vi "MainV2.vi"() -> ()   [LabVIEW 2010]
uses:
  <vilib>/Instr/_visa.llb/VISA Set IO Buffer Mask.ctl
  <vilib>/Instr/_visa.llb/VISA Flush IO Buffer Mask.ctl
  GlobalVar.vi
  <vilib>/Instr/_visa.llb/VISA Configure Serial Port (Instr).vi
  <vilib>/Utility/file.llb/Write To Spreadsheet File (string).vi
panel:
  out "Index Tableau":i32
  out "sortie d'erreur 3":errorcluster caption="sortie d'erreur"
  out "sortie d'erreur 2":errorcluster caption="sortie d'erreur"
  out "sortie d'erreur":errorcluster
  in  "Send":bool
  in  "Data to send":sgl
  in  "Command type":u16(ring)=129 items=["COEF_COURANT_2_INF"=36, "COEF_COURANT_2_CON"=164, "COEF_COURANT_1_INF"=35, "COEF_COURANT_1_CON"=163, "COEF_HYSTERISIS_SECURITE_INF"=34, "POURCENT_SECURITE_MOTEUR_INF"=33, "VITESSE_TROTTOIR_MAX_INF"=32, "DEMARRAGE_DELAI_EQUILIBRE_INF"=31, "DEMARRAGE_TOL_GUIDON_INF"=30, "DEMARRAGE_TOL_ANGLE_INF"=29, "LIMITE_DISTANCE_UTILISATEUR_INF"=28, "GUIDONMAX_INF"=27, "ACCELERATION_COEF_FILTRE_INF"=26, "COEF_KALMAN_INF"=25, "PRINC_DIR_INF"=24, "PRINC_PID_D_INF"=23, "PRINC_PID_K_INF"=22, "COEF_HYSTERISIS_SECURITE_CON"=162, "POURCENT_SECURITE_MOTEUR_CON"=161, "VITESSE_TROTTOIR_MAX_CON"=160, "DEMARRAGE_DELAI_EQUILIBRE_CON"=159, "DEMARRAGE_TOL_GUIDON_CON"=158, "DEMARRAGE_TOL_ANGLE_CON"=157, "LIMITE_DISTANCE_UTILISATEUR_CON"=156, "GUIDONMAX_CON"=155, "ACCELERATION_COEF_FILTRE_CON"=154, "COEF_KALMAN_CON"=153, "PRINC_DIR_CON"=152, "PRINC_PID_D_CON"=151, "PRINC_PID_K_CON"=150, "ENREGISTER_DEMARRAGE"=149, "CHARGER_DEMARRAGE"=148, "ENREGISTRER_ASSERVISSEMENT"=147, "CHARGER_ASSERVISSEMENT"=146, "ENREGISTRER_VITESSE"=145, "CHARGER_VITESSE"=144, "DEMANDE_COEFFICIENTS"=137, "VERBOSE_INF"=8, "VERBOSE_CON"=136, "ETAT"=1, "STOP"=131, "DEPART"=130, "TEST_COM"=129]
  out "LongToSend":u8
  out "TypeToSend":u8
  out "DataToSend":u8[](array[numeric])
  out "Frequency":dbl
  out "Enum":T1(ring)
  out "error":errorcluster
  out "error Connexion":errorcluster
  out "Stop main loop":bool
  in  "stop":bool
  in  "Tab Control":T2(tab)
  out "Reception":string
  in  "Comm_BaudRate":u32=9600 caption="Baud rate"
  in  "Comm_PortComm":refnum<visa-resource-name>="COM33" caption="Communication Port"
  in  "timeout (10sec)":u32=10000
  in  "Con_RefreshIntensity":bool caption="Bouton OK 12"
  in  "Con_RefreshRightTorque":bool caption="Bouton OK 12"
  out "Con_XYIntensity":cluster{"Y":dbl[], "Y":dbl[]}[](graph) caption="Intensity"
  out "Con_XYRightTorque":cluster{"Y":dbl[], "Y":dbl[]}[](graph) caption="Motor right Torque"
  in  "Con_RefreshLeftTorque":bool caption="Bouton OK 12"
  out "Con_XYLeftTorque":cluster{"Y":dbl[], "Y":dbl[]}[](graph) caption="Motor left Torque"
  out "Con_IntensityMax":bool caption="Max Intensity"
  out "Con_Intensity":string[][](array[string]) caption="Intensity (A)"
  out "Con_MotorRightTorque":string[][](array[string]) caption="Motor right Torque (N.m)"
  out "Con_MotorLeftTorque":string[][](array[string]) caption="Motor left Torque (N.m)"
  in  "Ana_RefreshBattery":bool caption="Bouton OK 12"
  out "Ana_XYBattery":cluster{"Y":dbl[], "Y":dbl[]}[](graph) caption="Motor left Torque"
  in  "Ana_RefreshHandlebar":bool caption="Bouton OK 12"
  out "Ana_XYHandlebar":cluster{"Y":dbl[], "Y":dbl[]}[](graph) caption="Motor left Torque"
  out "Ana_Battery":string[][](array[string]) caption="Battery"
  out "Ana_Handlebar":string[][](array[string]) caption="Handlebar"
  in  "Inc_RefreshAcceleration":bool caption="Bouton OK 12"
  out "Inc_XYAcceleration":cluster{"Y":dbl[], "Y":dbl[]}[](graph) caption="Motor left Torque"
  in  "Inc_RefreshVelocityRightMotor":bool caption="Bouton OK 12"
  out "Inc_XYVelocityRightMotor":cluster{"Y":dbl[], "Y":dbl[]}[](graph) caption="Motor left Torque"
  in  "Inc_RefreshVelocityLeftMotor":bool caption="Bouton OK 12"
  out "Inc_XYVelocityLeftMotor":cluster{"Y":dbl[], "Y":dbl[]}[](graph) caption="Motor left Torque"
  out "Inc_Acceleration":string[][](array[string]) caption="Acceleration"
  out "Inc_VelocityRightMotor":string[][](array[string]) caption="Velocity Right motor"
  out "Inc_VelocityLeftMotor":string[][](array[string]) caption="Velocity left motor"
  out "Oth_XYAngularVelocity":cluster{"Y":dbl[], "Y":dbl[]}[](graph) caption="Motor left Torque"
  out "Oth_XYDistance":cluster{"Y":dbl[], "Y":dbl[]}[](graph) caption="Motor left Torque"
  out "Oth_XYAngle":cluster{"Y":dbl[], "Y":dbl[]}[](graph) caption="Motor left Torque"
  in  "Oth_RefreshAngularVelocity":bool caption="Bouton OK 12"
  in  "Oth_RefreshDistance":bool caption="Bouton OK 12"
  in  "Oth_RefreshAngle":bool caption="Bouton OK 12"
  out "Other_AngularVelocity":string[][](array[string]) caption="Angular velocity"
  out "Other_Distance":string[][](array[string]) caption="Distance"
  out "Other_Angle":string[][](array[string]) caption="Angle"
  in  "Analyse_Send":bool
  in  "Analyse_Time":dbl caption="Time"
  in  "Analyse_Step":dbl caption="Step"
  in  "Analyse_LeftOrRight":bool caption="Booléen"
  out "Analyse_XYTorque":cluster{"Y":dbl[], "Y":dbl[]}[](graph) caption="Motor Torque command"
  out "Analyse_MotorTorque":string[][](array[string]) caption="Motor  Torque (N.m)"
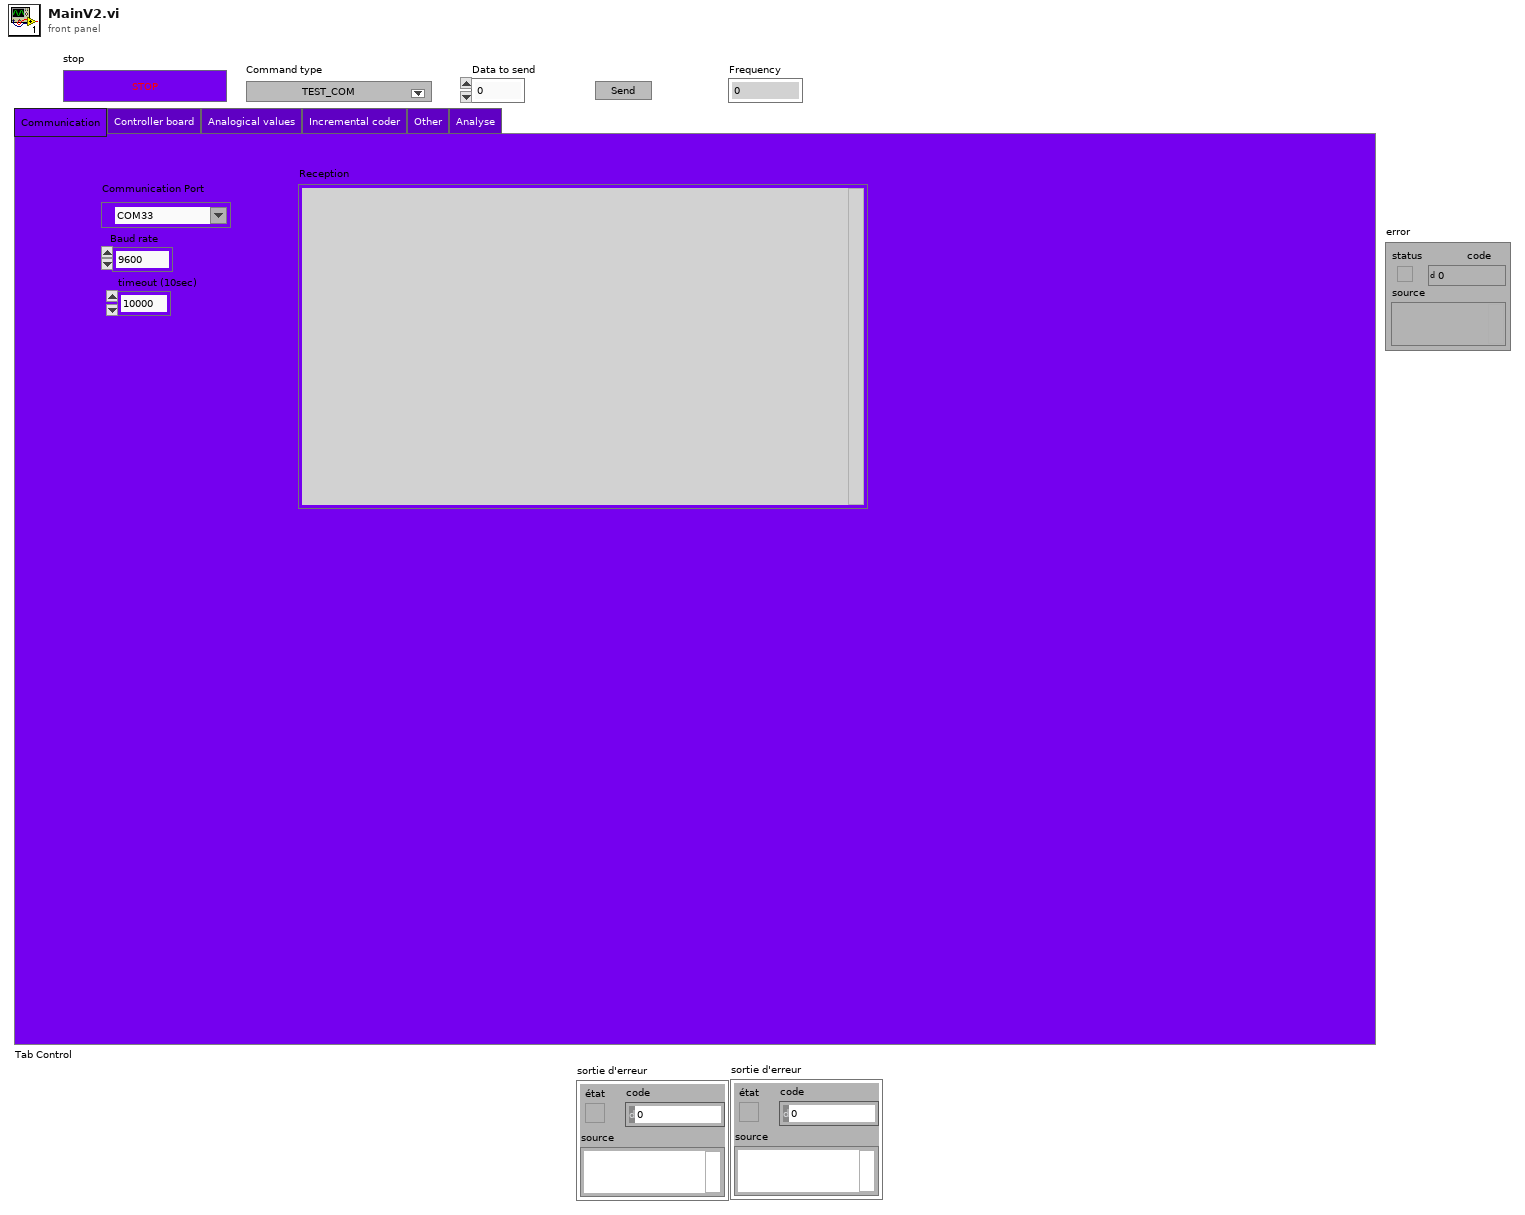
[diagram p1: front panel]
types:
  T1 = enum16{"Send_Instruction", "Con_RefreshLeftTorque", "Con_RefreshRightTorque", "Con_RefreshIntensity", "Ana_RefreshBattery", "Ana_RefreshHandlebar", "Inc_RefreshVelocityLeftMotor", "Inc_RefreshVelocityRightMotor", "Inc_RefreshAcceleration", "SendAnalysis", "Oth_RefreshAngle", "Oth_RefreshDistance", "Oth_RefreshAngularVelocity", "Waiting"}
  T2 = enum32{"Communication", "Controller board", "Analogical values", "Incremental coder", "Other", "Analyse"}
  T3 = typedef "VISA Set IO Buffer Mask.ctl" = u16
  T4 = typedef "VISA Flush IO Buffer Mask.ctl" = u16
  T5 = enum16{"Send_Instruction", "Con_RefreshLeftTorque", "Con_RefreshRightTorque", "Con_RefreshIntensity", "Ana_RefreshBattery", "Ana_RefreshHandlebar", "Inc_RefreshVelocityLeftMotor", "Inc_RefreshVelocityRightMotor", "Inc_RefreshAcceleration", "SendAnalysis", "Oth_RefreshAngle", "Oth_RefreshDistance", "Oth_RefreshAgularVelocity", "Waiting"}
  T6 = enum16{"Send_Instruction", "Con_RefreshLeftTorque", "Con_RefreshRightTorque", "Con_RefreshIntensity", "Ana_RefreshBattery", "Ana_RefreshHandlebar", "Inc_RefreshVelocityLeftMotor", "Inc_RefreshVelocityRightMotor", "Inc_RefreshAcceleration", "SendAnalysis", "Waiting"}
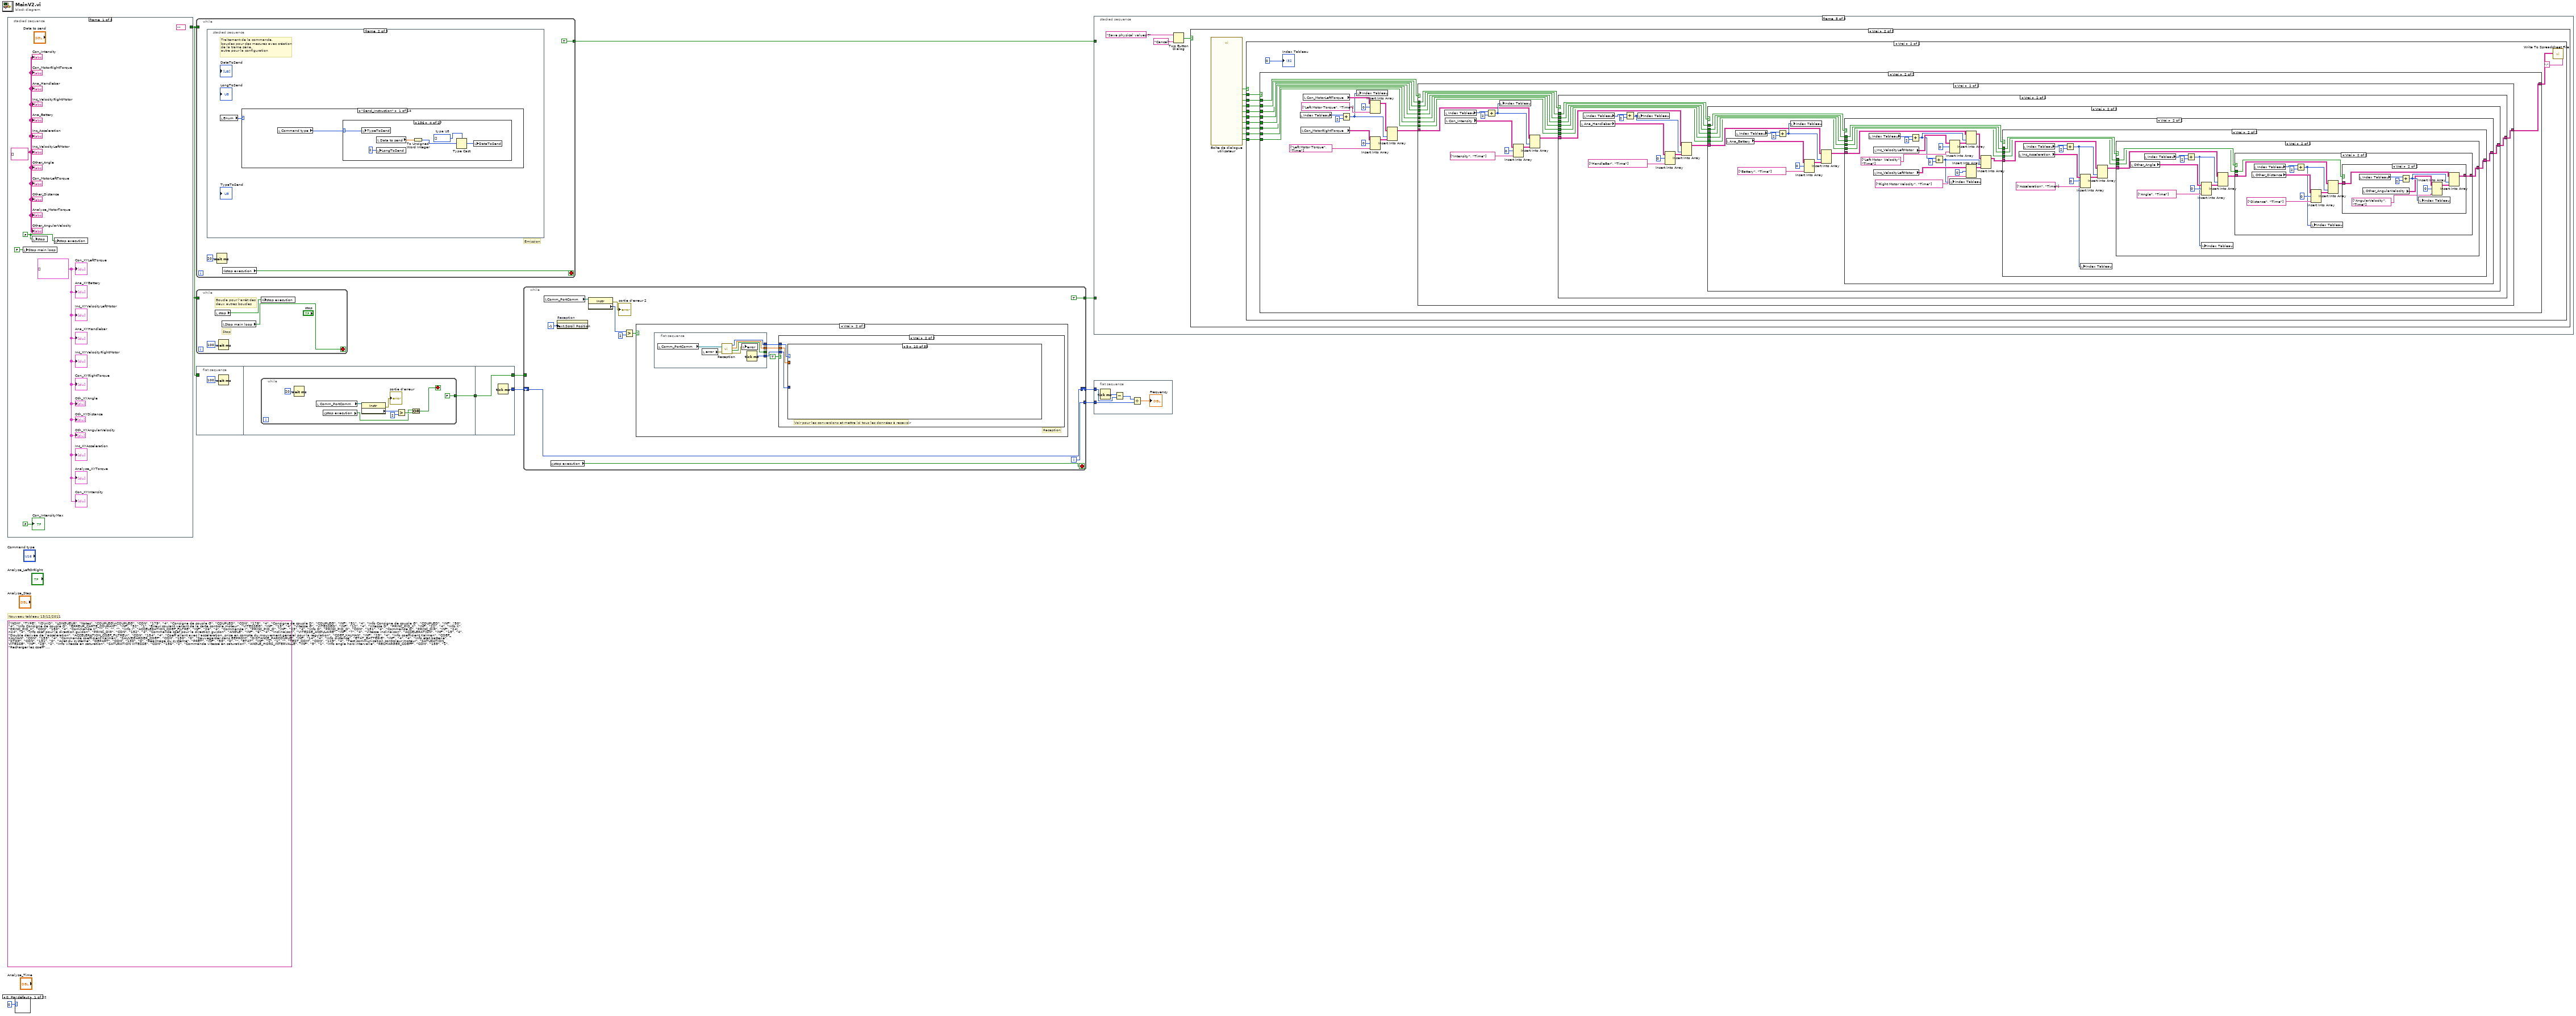
[diagram p0: block diagram]
diagram:
  (unwired) string[][] [["NOM", "TYPE", "ID\nID", "LONGUEUR", "Notes"], ["COUPLEG\nCOUPLEG", "CON", "179", "4", "Consigne de couple G"], ["COUPLED", "CON", "178", "4", "Consigne de couple D"], ["COUPLEG", "INF", "51", "4", "Info Consigne de couple G"], ["COUPLED", "INF", "50", "4", "Info Consigne de couple D"], ["ERREUR_CARTE_COURANT", "INF", "52", "1", "Erreur courant venant de la carte contrôle moteur"], ["VITESSEG", "INF", "13", "4", "Vitesse G"], ["VITESSED", "INF", "12", "4", "Vitesse D"], ["PRINC_PID_K", "INF", "22", "4", "Info K"], ["PRINC_PID_K", "CON", "150", "4", "Commande K"], ["", "", "", "", "Info I"], ["ACCELERATION_COEF_FILTRE", "INF", "26", "4", "Commande I"], ["PRINC_PID_D", "INF", "23", "4", "Info D"], ["PRINC_PID_D", "CON", "151", "4", "Commande D"], ["PRINC_DIR", "INF", "24\n24", "4", "Info coef pour la direction guidon"], ["PRINC_DIR", "CON", "152", "4", "Commande coef pour la direction guidon"], ["ANGLE", "INF", "6", "4", "Inclinaison"], ["VITESSE_ANGULAIRE", "INF", "7", "4", "Vitesse inclinaison"], ["ACCELERATION", "INF", "15", "4", "Double dérivée de l'accélération"], ["ACCELERATION_COEF_FILTRE\n", "CON", "154", "4", "Coeff allant avec l'accélération, prise en compte du mouvement général pour la régulation"], ["COEF_KALMAN", "INF", "25", "4", "Info coefficient Kalman"], ["COEF_KALMAN", "CON", "153", "4", "Commande coefficient Kalman"], ["SAUVEGARDER_COEF", "CON", "150", "0", "Sauvegarder dans EEPROM"], ["DISTANCE_PARCOURUE", "INF", "14", "4", "Info distance"], ["ETAT_BATTERIE", "INF", "4", "4", "Info etat batterie"], ["STOP", "CON", "131", "0", "Arret du système"], ["DEPART", "CON", "130", "0", "Réarmage du système"], ["PRET", "INF", "53", "0", ""], ["ETAT", "INF", "1", "1", ""], ["TEST_COM", "CON", "129", "4", "Test communication controleur moteur"], ["SATURATION_VITESSE", "INF", "28", "2", "Info vitesse en saturation"], ["SATURATION VITESSE", "CON", "156", "2", "Commande vitesse en saturation"], ["ANGLE_HORS_INTERVALLE", "INF", "5", "1", "Info angle hors intervalle"], ["RECHARGER_COEFF", "CON", "159", "1", "Recharger les coeff"], ["VERBOSE", "INF", "8", "2", ""], ["VERBOSE", "CON", "136", "2", ""], ["DEMANDE_COEFFICIENTS", "CON", "137", "1", ""], ["CHARGER_VITESSE", "CON", "144", "0", ""], ["ENREGISTRER_VITESSE", "CON", "145", "0", ""], ["CHARGER_ASSERVISSEMENT", "CON", "146", "0", ""], ["ENREGISTRER_ASSERVISSEMENT", "CON", "147", "0", ""], ["CHARGER_DEMARRAGE", "CON", "148", "0", ""], ["ENREGISTRER_DEMARRAGE", "CON", "149", "0", ""], ["GUIDONMAX", "INF", "27", "4", ""], ["LIMITE_DISTANCE_UTILISATEUR", "INF", "28", "4", ""], ["DEMARRAGE_TOL_ANGLE", "INF", "29", "4", ""], ["DEMARRAGE_TOL_GUIDON", "INF", "30", "4", ""], ["DEMARRAGE_DELAI_EQUILIBRE", "INF", "31", "4", ""], ["VITESSE_TROTTOIR_MAX", "INF", "32", "4", ""], ["POURCENT_SECURITE_MOTEUR", "INF", "33", "4", ""], ["COEF_HYSTERESIS_SECURITE", "INF", "34", "4", ""], ["COEF_COURANT_1", "CON", "163", "4", ""], ["COEF_COURANT_1", "INF", "35", "4", ""], ["COEF_COURANT_2", "CON", "164", "4", ""], ["COEF_COURANT_2", "INF", "36", "4", ""]]
  # "Nouveau tableau 13/12/2011"
  n1 = stacked-sequence {
    tunnel: [_ _ TRUE] -> w4
    frame #0 {
      (unwired) "" ("Spe_Liste")
      w11 = cluster{"Y":dbl[], "Y":dbl[]}[] [] ("Ana_XYHandlebar 3")
      w10 = string[][] [] ("Velocity motor left")
      w13 = FALSE ("Comm_LEDTest")
      n2 = local write "Stop main loop"(FALSE ("Stop main loop")) -> ()
      n3 = local write "stop"(w13) -> ()
      n4 = global write "GlobalVar.vi" "stop execution"(w13) -> ()
      "Con_IntensityMax" <- FALSE ("Con_IntensityMax")
      "Inc_Acceleration" <- w10
      "Other_Angle" <- w10
      "Other_Distance" <- w10
      "Ana_XYHandlebar" <- w11
      "Ana_XYBattery" <- w11
      "Inc_XYVelocityLeftMotor" <- w11
      "Inc_XYVelocityRightMotor" <- w11
      "Inc_XYAcceleration" <- w11
      "Con_MotorLeftTorque" <- w10
      "Con_MotorRightTorque" <- w10
      "Con_Intensity" <- w10
      "Inc_VelocityLeftMotor" <- w10
      "Inc_VelocityRightMotor" <- w10
      "Ana_Handlebar" <- w10
      "Ana_Battery" <- w10
      "Con_XYRightTorque" <- w11
      "Con_XYIntensity" <- w11
      "Con_XYLeftTorque" <- w11
      "Other_AngularVelocity" <- w10
      "Oth_XYAngle" <- w11
      "Oth_XYDistance" <- w11
      "Oth_XYAngularVelocity" <- w11
      "Analyse_XYTorque" <- w11
      "Analyse_MotorTorque" <- w10
    }
    frame #1 {
      w18 = T3 48 items=["Buffer d'entrées (E/S)"=16, "Buffer de sorties (E/S)"=32, "Buffer d'entrées et de sorties (E/S)"=48] ("Mask")
      w22 = T4 16 items=["Vider le buffer d'entrées"=16, "Écrire le buffer de sorties sur le périphérique"=32, "Vider le buffer d'entrées (Pas d'E/S)"=64, "Vider le buffer de sorties"=128] ("Mask")
      w25 = u16 0 items=["None"=0, "XON/XOFF"=1, "RTS/CTS"=2, "DTR/DSR"=4] ("flow control")
      w26 = u16 10 items=["1.0"=10, "1.5"=15, "2.0"=20] ("stop bits")
      w28 = u16 0 items=["None", "Odd", "Even", "Mark", "Space"] ("parity")
      # "Initial"
      n5 = local write "Tab Control"(T2."Communication" ("Tab Control")) -> ()
      n6 = call-poly "VISA Configure Serial Port"("VISA resource name"="Comm_PortComm", "timeout (10sec)"="timeout (10sec)", "baud rate (9600)"="Comm_BaudRate", "data bits (8)"=u16 8 ("data bits"), "parity (0:none)"=w28, "stop bits (10: 1 bit)"=w26, "flow control (0:none)"=w25) -> ("VISA resource name out"=w23:refnum<visa-resource-name>, "error out"=w20:errorcluster)  [unwired: 2 in, 5 out]
      "error Connexion" <- w20
      "error" <- w20
      n7 = VISA Set I/O Buffer Size(VISA resource name=w23, mask (16)=w18, size (4096)=u32 524288 ("taille (4096)"), error in (no error)=w20) -> (VISA resource name out=w21:refnum<visa-resource-name>, error out=w19:errorcluster)
      n8 = VISA Flush I/O Buffer(VISA resource name=w21, mask (16)=w22, error in (no error)=w19) -> ()  [unwired: 2 out]
      "Reception" <- "" ("Reception")
    }
    frame #2 {
      # "OK Initialisation"
    }
  }
  n9 = case shown="0, Par défaut" 0 {
    frame 0, Default {
    }
    frame 10 {
    }
    frame 11 {
    }
    frame 12 {
    }
    frame 13 {
    }
    frame 14 {
    }
    frame 15 {
    }
    frame 16 {
    }
    frame 17 {
    }
    frame 18 {
    }
    frame 19 {
    }
    frame 20 {
    }
    frame 21 {
    }
    frame 22 {
    }
    frame 23 {
    }
    frame 24 {
    }
    frame 25 {
    }
    frame 26 {
    }
    frame 27 {
    }
    frame 28 {
    }
    frame 29 {
    }
    frame 30 {
    }
  }
  n10 = while {
    tunnel: w4 -> [_]
    tunnel: [TRUE] -> w8
    stop <- w33 stop-if-true
    # "Emission"
    n11 = stacked-sequence {
      frame #0 {
        # "Detection de la commande\ndemandée"
        n12 = Build Array("Send", "Con_RefreshLeftTorque", "Con_RefreshRightTorque", "Con_RefreshIntensity", "Ana_RefreshBattery", "Ana_RefreshHandlebar", "Inc_RefreshVelocityLeftMotor", "Inc_RefreshVelocityRightMotor", "Inc_RefreshAcceleration", "Analyse_Send", "Oth_RefreshAngle", "Oth_RefreshDistance", "Oth_RefreshAngularVelocity") -> (w53:bool[])
        n13 = Search 1D Array(1D array=w53, element=TRUE) -> (index of element=w49:i32)  [unwired: 1 in]
        n14 = Equal?(x=w49, y=-1) -> (x = y?=w51:bool)
        n15 = case shown="Vrai" w51 {
          tunnel: [w54 T5."Waiting" ("Enum 2")] -> w50
          tunnel: w49 -> [w54 _]
          frame False {
          }
          frame True {
          }
        }
        "Enum" <- w50
      }
      frame #1 {
        # "Traitement de la commande,\nboucles pour des mesures avec création \nde la trame série,\nautre pour la configuration"
        n16 = local read "Enum"() -> (w56:T1)
        n17 = case shown="\"Send_Instruction\"" w56 {
          frame "Send_Instruction" {
            n18 = local read "Command type"() -> (w57:u16)
            n19 = case shown="136" w57 {
              selector: w57 -> [w62 w64 w69 w75 w79 w84 w89 w94 w99 w104 w109 w114 w119 w124 w129 w134 w139 w144 w149 w154 w159 w164 w169 w174 w179 w184 _]
              frame 129 {
                w60 = u8[] []  # type U8
                n20 = local write "TypeToSend"(w62) -> ()
                n21 = local write "LongToSend"(u8 4 ("LongToSend")) -> ()
                n22 = local read "Data to send"() -> (w58:sgl)
                n23 = Type Cast(type=w60, x=w58) -> (*(type *) &x=w59:u8[])
                n24 = local write "DataToSend"(w59) -> ()
              }
              frame 130 {
                w66 = u8[] []  # type U8
                n25 = local write "TypeToSend"(w64) -> ()
                n26 = local write "LongToSend"(u8 0 ("LongToSend")) -> ()
                n27 = local read "Data to send"() -> (w63:sgl)
                n28 = Type Cast(type=w66, x=w63) -> (*(type *) &x=w65:u8[])
                n29 = local write "DataToSend"(w65) -> ()
              }
              frame 131 {
                w71 = u8[] []  # type U8
                n30 = local write "TypeToSend"(w69) -> ()
                n31 = local write "LongToSend"(u8 0 ("LongToSend")) -> ()
                n32 = local read "Data to send"() -> (w68:sgl)
                n33 = Type Cast(type=w71, x=w68) -> (*(type *) &x=w70:u8[])
                n34 = local write "DataToSend"(w70) -> ()
              }
              frame 136 {
                w77 = u8[] []  # type U8
                n35 = local write "TypeToSend"(w75) -> ()
                n36 = local write "LongToSend"(u8 2 ("LongToSend")) -> ()
                n37 = local read "Data to send"() -> (w74:sgl)
                n38 = To Unsigned Word Integer(number=w74) -> (unsigned 16bit integer=w73:u16)
                n39 = Type Cast(type=w77, x=w73) -> (*(type *) &x=w76:u8[])
                n40 = local write "DataToSend"(w76) -> ()
              }
              frame 137 {
                w81 = u8[] []  # type U8
                n41 = local write "TypeToSend"(w79) -> ()
                n42 = local write "LongToSend"(u8 0 ("LongToSend")) -> ()
                n43 = local read "Data to send"() -> (w83:sgl)
                n44 = Type Cast(type=w81, x=w83) -> (*(type *) &x=w80:u8[])
                n45 = local write "DataToSend"(w80) -> ()
              }
              frame 144 {
                w86 = u8[] []  # type U8
                n46 = local write "TypeToSend"(w84) -> ()
                n47 = local write "LongToSend"(u8 0 ("LongToSend")) -> ()
                n48 = local read "Data to send"() -> (w88:sgl)
                n49 = Type Cast(type=w86, x=w88) -> (*(type *) &x=w85:u8[])
                n50 = local write "DataToSend"(w85) -> ()
              }
              frame 145 {
                w91 = u8[] []  # type U8
                n51 = local write "TypeToSend"(w89) -> ()
                n52 = local write "LongToSend"(u8 0 ("LongToSend")) -> ()
                n53 = local read "Data to send"() -> (w93:sgl)
                n54 = Type Cast(type=w91, x=w93) -> (*(type *) &x=w90:u8[])
                n55 = local write "DataToSend"(w90) -> ()
              }
              frame 146 {
                w96 = u8[] []  # type U8
                n56 = local write "TypeToSend"(w94) -> ()
                n57 = local write "LongToSend"(u8 0 ("LongToSend")) -> ()
                n58 = local read "Data to send"() -> (w98:sgl)
                n59 = Type Cast(type=w96, x=w98) -> (*(type *) &x=w95:u8[])
                n60 = local write "DataToSend"(w95) -> ()
              }
              frame 147 {
                w101 = u8[] []  # type U8
                n61 = local write "TypeToSend"(w99) -> ()
                n62 = local write "LongToSend"(u8 0 ("LongToSend")) -> ()
                n63 = local read "Data to send"() -> (w103:sgl)
                n64 = Type Cast(type=w101, x=w103) -> (*(type *) &x=w100:u8[])
                n65 = local write "DataToSend"(w100) -> ()
              }
              frame 148 {
                w106 = u8[] []  # type U8
                n66 = local write "TypeToSend"(w104) -> ()
                n67 = local write "LongToSend"(u8 0 ("LongToSend")) -> ()
                n68 = local read "Data to send"() -> (w108:sgl)
                n69 = Type Cast(type=w106, x=w108) -> (*(type *) &x=w105:u8[])
                n70 = local write "DataToSend"(w105) -> ()
              }
              frame 149 {
                w111 = u8[] []  # type U8
                n71 = local write "TypeToSend"(w109) -> ()
                n72 = local write "LongToSend"(u8 0 ("LongToSend")) -> ()
                n73 = local read "Data to send"() -> (w113:sgl)
                n74 = Type Cast(type=w111, x=w113) -> (*(type *) &x=w110:u8[])
                n75 = local write "DataToSend"(w110) -> ()
              }
              frame 150 {
                w116 = u8[] []  # type U8
                n76 = local write "TypeToSend"(w114) -> ()
                n77 = local write "LongToSend"(u8 4 ("LongToSend")) -> ()
                n78 = local read "Data to send"() -> (w118:sgl)
                n79 = Type Cast(type=w116, x=w118) -> (*(type *) &x=w115:u8[])
                n80 = local write "DataToSend"(w115) -> ()
              }
              frame 151 {
                w121 = u8[] []  # type U8
                n81 = local write "TypeToSend"(w119) -> ()
                n82 = local write "LongToSend"(u8 4 ("LongToSend")) -> ()
                n83 = local read "Data to send"() -> (w123:sgl)
                n84 = Type Cast(type=w121, x=w123) -> (*(type *) &x=w120:u8[])
                n85 = local write "DataToSend"(w120) -> ()
              }
              frame 152 {
                w126 = u8[] []  # type U8
                n86 = local write "TypeToSend"(w124) -> ()
                n87 = local write "LongToSend"(u8 4 ("LongToSend")) -> ()
                n88 = local read "Data to send"() -> (w128:sgl)
                n89 = Type Cast(type=w126, x=w128) -> (*(type *) &x=w125:u8[])
                n90 = local write "DataToSend"(w125) -> ()
              }
              frame 153 {
                w131 = u8[] []  # type U8
                n91 = local write "TypeToSend"(w129) -> ()
                n92 = local write "LongToSend"(u8 4 ("LongToSend")) -> ()
                n93 = local read "Data to send"() -> (w133:sgl)
                n94 = Type Cast(type=w131, x=w133) -> (*(type *) &x=w130:u8[])
                n95 = local write "DataToSend"(w130) -> ()
              }
              frame 154 {
                w136 = u8[] []  # type U8
                n96 = local write "TypeToSend"(w134) -> ()
                n97 = local write "LongToSend"(u8 4 ("LongToSend")) -> ()
                n98 = local read "Data to send"() -> (w138:sgl)
                n99 = Type Cast(type=w136, x=w138) -> (*(type *) &x=w135:u8[])
                n100 = local write "DataToSend"(w135) -> ()
              }
              frame 155 {
                w141 = u8[] []  # type U8
                n101 = local write "TypeToSend"(w139) -> ()
                n102 = local write "LongToSend"(u8 4 ("LongToSend")) -> ()
                n103 = local read "Data to send"() -> (w143:sgl)
                n104 = Type Cast(type=w141, x=w143) -> (*(type *) &x=w140:u8[])
                n105 = local write "DataToSend"(w140) -> ()
              }
              frame 156 {
                w146 = u8[] []  # type U8
                n106 = local write "TypeToSend"(w144) -> ()
                n107 = local write "LongToSend"(u8 4 ("LongToSend")) -> ()
                n108 = local read "Data to send"() -> (w148:sgl)
                n109 = Type Cast(type=w146, x=w148) -> (*(type *) &x=w145:u8[])
                n110 = local write "DataToSend"(w145) -> ()
              }
              frame 157 {
                w151 = u8[] []  # type U8
                n111 = local write "TypeToSend"(w149) -> ()
                n112 = local write "LongToSend"(u8 4 ("LongToSend")) -> ()
                n113 = local read "Data to send"() -> (w153:sgl)
                n114 = Type Cast(type=w151, x=w153) -> (*(type *) &x=w150:u8[])
                n115 = local write "DataToSend"(w150) -> ()
              }
              frame 158 {
                w156 = u8[] []  # type U8
                n116 = local write "TypeToSend"(w154) -> ()
                n117 = local write "LongToSend"(u8 4 ("LongToSend")) -> ()
                n118 = local read "Data to send"() -> (w158:sgl)
                n119 = Type Cast(type=w156, x=w158) -> (*(type *) &x=w155:u8[])
                n120 = local write "DataToSend"(w155) -> ()
              }
              frame 159 {
                w161 = u8[] []  # type U8
                n121 = local write "TypeToSend"(w159) -> ()
                n122 = local write "LongToSend"(u8 4 ("LongToSend")) -> ()
                n123 = local read "Data to send"() -> (w163:sgl)
                n124 = Type Cast(type=w161, x=w163) -> (*(type *) &x=w160:u8[])
                n125 = local write "DataToSend"(w160) -> ()
              }
              frame 160 {
                w166 = u8[] []  # type U8
                n126 = local write "TypeToSend"(w164) -> ()
                n127 = local write "LongToSend"(u8 4 ("LongToSend")) -> ()
                n128 = local read "Data to send"() -> (w168:sgl)
                n129 = Type Cast(type=w166, x=w168) -> (*(type *) &x=w165:u8[])
                n130 = local write "DataToSend"(w165) -> ()
              }
              frame 161 {
                w171 = u8[] []  # type U8
                n131 = local write "TypeToSend"(w169) -> ()
                n132 = local write "LongToSend"(u8 4 ("LongToSend")) -> ()
                n133 = local read "Data to send"() -> (w173:sgl)
                n134 = Type Cast(type=w171, x=w173) -> (*(type *) &x=w170:u8[])
                n135 = local write "DataToSend"(w170) -> ()
              }
              frame 162 {
                w176 = u8[] []  # type U8
                n136 = local write "TypeToSend"(w174) -> ()
                n137 = local write "LongToSend"(u8 4 ("LongToSend")) -> ()
                n138 = local read "Data to send"() -> (w178:sgl)
                n139 = Type Cast(type=w176, x=w178) -> (*(type *) &x=w175:u8[])
                n140 = local write "DataToSend"(w175) -> ()
              }
              frame 163 {
                w181 = u8[] []  # type U8
                n141 = local write "TypeToSend"(w179) -> ()
                n142 = local write "LongToSend"(u8 4 ("LongToSend")) -> ()
                n143 = local read "Data to send"() -> (w183:sgl)
                n144 = Type Cast(type=w181, x=w183) -> (*(type *) &x=w180:u8[])
                n145 = local write "DataToSend"(w180) -> ()
              }
              frame 164 {
                w186 = u8[] []  # type U8
                n146 = local write "TypeToSend"(w184) -> ()
                n147 = local write "LongToSend"(u8 4 ("LongToSend")) -> ()
                n148 = local read "Data to send"() -> (w188:sgl)
                n149 = Type Cast(type=w186, x=w188) -> (*(type *) &x=w185:u8[])
                n150 = local write "DataToSend"(w185) -> ()
              }
              frame 0, Default {
                n151 = One Button Dialog(message="No transmission.") -> ()  [unwired: 1 in, 1 out]
              }
            }
          }
          frame "Con_RefreshRightTorque" {
            n152 = local read "Con_MotorRightTorque"() -> (w191:string[][])
            n153 = call "TableToXYGraph.vi"("Input Table"=w191) -> ("XY Graph"=w190:cluster{"Y":dbl[], "Y":dbl[]}[])
            n154 = local write "Con_XYRightTorque"(w190) -> ()
          }
          frame "Con_RefreshIntensity" {
            n155 = local read "Con_Intensity"() -> (w193:string[][])
            n156 = call "TableToXYGraph.vi"("Input Table"=w193) -> ("XY Graph"=w192:cluster{"Y":dbl[], "Y":dbl[]}[])
            n157 = local write "Con_XYIntensity"(w192) -> ()
          }
          frame "Ana_RefreshBattery" {
            n158 = local read "Ana_Battery"() -> (w195:string[][])
            n159 = call "TableToXYGraph.vi"("Input Table"=w195) -> ("XY Graph"=w194:cluster{"Y":dbl[], "Y":dbl[]}[])
            n160 = local write "Ana_XYBattery"(w194) -> ()
          }
          frame "Ana_RefreshHandlebar" {
            n161 = local read "Ana_Handlebar"() -> (w197:string[][])
            n162 = call "TableToXYGraph.vi"("Input Table"=w197) -> ("XY Graph"=w196:cluster{"Y":dbl[], "Y":dbl[]}[])
            n163 = local write "Ana_XYHandlebar"(w196) -> ()
          }
          frame "Inc_RefreshVelocityLeftMotor" {
            n164 = local read "Inc_VelocityLeftMotor"() -> (w199:string[][])
            n165 = call "TableToXYGraph.vi"("Input Table"=w199) -> ("XY Graph"=w198:cluster{"Y":dbl[], "Y":dbl[]}[])
            n166 = local write "Inc_XYVelocityLeftMotor"(w198) -> ()
          }
          frame "Inc_RefreshVelocityRightMotor" {
            n167 = local read "Inc_VelocityRightMotor"() -> (w201:string[][])
            n168 = call "TableToXYGraph.vi"("Input Table"=w201) -> ("XY Graph"=w200:cluster{"Y":dbl[], "Y":dbl[]}[])
            n169 = local write "Inc_XYVelocityRightMotor"(w200) -> ()
          }
          frame "Inc_RefreshAcceleration" {
            n170 = local read "Inc_Acceleration"() -> (w203:string[][])
            n171 = call "TableToXYGraph.vi"("Input Table"=w203) -> ("XY Graph"=w202:cluster{"Y":dbl[], "Y":dbl[]}[])
            n172 = local write "Inc_XYAcceleration"(w202) -> ()
          }
          frame "SendAnalysis" {
            n173 = One Button Dialog(message="Not available.") -> ()  [unwired: 1 in, 1 out]
          }
          frame "Con_RefreshLeftTorque" {
            n174 = local read "Con_MotorLeftTorque"() -> (w206:string[][])
            n175 = call "TableToXYGraph.vi"("Input Table"=w206) -> ("XY Graph"=w205:cluster{"Y":dbl[], "Y":dbl[]}[])
            n176 = local write "Con_XYLeftTorque"(w205) -> ()
          }
          frame "Oth_RefreshAngle" {
            n177 = local read "Other_Angle"() -> (w208:string[][])
            n178 = call "TableToXYGraph.vi"("Input Table"=w208) -> ("XY Graph"=w207:cluster{"Y":dbl[], "Y":dbl[]}[])
            n179 = local write "Oth_XYAngle"(w207) -> ()
          }
          frame "Oth_RefreshDistance" {
            n180 = local read "Other_Distance"() -> (w210:string[][])
            n181 = call "TableToXYGraph.vi"("Input Table"=w210) -> ("XY Graph"=w209:cluster{"Y":dbl[], "Y":dbl[]}[])
            n182 = local write "Oth_XYDistance"(w209) -> ()
          }
          frame "Oth_RefreshAngularVelocity" {
            n183 = local read "Other_AngularVelocity"() -> (w212:string[][])
            n184 = call "TableToXYGraph.vi"("Input Table"=w212) -> ("XY Graph"=w211:cluster{"Y":dbl[], "Y":dbl[]}[])
            n185 = local write "Oth_XYAngularVelocity"(w211) -> ()
          }
          frame "Waiting", Default {
            # "nop"
          }
        }
      }
      frame #2 {
        n186 = local read "Enum"() -> (w215:T1)
        n187 = Equal?(x=w215, y=T6."Send_Instruction") -> (x = y?=w213:bool)
        n188 = case shown="Faux" w213 {
          frame False {
          }
          frame True {
            # "Envoyer la trame"
            n189 = local read "TypeToSend"() -> (w217:u8)
            n190 = local read "DataToSend"() -> (w218:u8[])
            n191 = local read "Comm_PortComm"() -> (w220:refnum<visa-resource-name>)
            n192 = local read "LongToSend"() -> (w216:u8)
            n193 = call "Send.vi"("Nom de ressource VISA"=w220, "tableau d'octets non signés"=w218, "Type"=w217, "Long_Data"=w216) -> ("sortie d'erreur"=w219:errorcluster)  [unwired: 1 in, 1 out]
            n194 = local write "error"(w219) -> ()
          }
        }
      }
    }
    n195 = Wait (ms)(milliseconds to wait=u32 20 ("attente (ms)")) -> ()  [unwired: 1 out]
    n196 = global read "GlobalVar.vi" "stop execution"() -> (w33:bool)
  }
  n197 = while {
    tunnel: w4 -> [_]
    stop <- w222 stop-if-true
    # "Boucle pour l'arrêt des \ndeux autres boucles"
    # "Stop"
    n198 = local read "stop"() -> (w223:bool)
    n199 = Wait (ms)(milliseconds to wait=u32 100) -> ()  [unwired: 1 out]
    n200 = local read "Stop main loop"() -> (w222:bool)
    n201 = global write "GlobalVar.vi" "stop execution"(w223) -> ()
  }
  n202 = flat-sequence {
    tunnel: w4 -> [_]
    tunnel: [w225] -> w3
    tunnel: [w236] -> w5
    tunnel: w3 -> [w236]
    tunnel: [w235] -> w2
    frame #0 {
      n203 = Wait (ms)(milliseconds to wait=u32 100 ("attente (ms)")) -> ()  [unwired: 1 out]
    }
    frame #1 {
      n204 = while {
        tunnel: [FALSE] -> w225
        stop <- w227 stop-if-true
        n205 = Wait (ms)(milliseconds to wait=u32 20 ("attente (ms)")) -> ()  [unwired: 1 out]
        n206 = local read "Comm_PortComm"() -> (w234:refnum<visa-resource-name>)
        n207 = global read "GlobalVar.vi" "stop execution"() -> (w228:bool)
        n208 = property class="Instr"(reference=w234) -> (error out=→"sortie d'erreur":errorcluster, "Serial Settings:Number of Bytes at Serial Port"=w233:u32)  [unwired: 1 in, 1 out]
        n209 = Greater?(x=w233, y=u32 2) -> (0:w231:bool)
        n210 = Or(x=w228, y=w231) -> (x .or. y?=w227:bool)
      }
    }
    frame #2 {
      n211 = Tick Count (ms)() -> (millisecond timer value=w235:u32)
    }
  }
  n212 = while {
    tunnel: [TRUE] -> w9
    tunnel: [w244] -> w6
    tunnel: w5 -> [_]
    shift-right: [w243] -> w1
    shift-left: w2 -> [w243]
    i -> [w244]
    stop <- w245 stop-if-true
    n213 = local read "Comm_PortComm"() -> (w242:refnum<visa-resource-name>)
    n214 = global read "GlobalVar.vi" "stop execution"() -> (w245:bool)
    n215 = property on="Reception" class="Ch"("Text.Scroll Position"=-1) -> ()  [unwired: 2 in, 2 out]
    n216 = property class="Instr"(reference=w242) -> (error out=→"sortie d'erreur 2":errorcluster, "Serial Settings:Number of Bytes at Serial Port"=w241:u32)  [unwired: 1 in, 1 out]
    n217 = Greater?(x=w241, y=u32 2) -> (0:w240:bool)
    n218 = case shown="Vrai" w240 {
      frame False {
      }
      frame True {
        # "Reception"
        n219 = flat-sequence {
          tunnel: [w255] -> _
          tunnel: [w254] -> w250
          tunnel: [w253] -> w249
          tunnel: [w252] -> w248
          frame #0 {
            n220 = local read "Comm_PortComm"() -> (w257:refnum<visa-resource-name>)
            n221 = local read "error"() -> (w256:errorcluster)
            n222 = call "Reception.vi"("entrée d'erreur (pas d'erreur)"=w256, "Nom de ressource VISA"=w257) -> ("Sortie d'erreur"=w251:errorcluster, "Checksum OK?"=w255:bool, "Data"=w253:sgl, "ID byte"=w254:i32)
            n223 = local write "error"(w251) -> ()
            n224 = Tick Count (ms)() -> (millisecond timer value=w252:u32)
          }
        }
        n225 = case shown="Vrai" TRUE {
          tunnel: w250 -> [_ w259]
          tunnel: w249 -> [_ w258]
          tunnel: w248 -> [_ w260]
          frame False {
          }
          frame True {
            # "Voir pour les conversions et mettre ici tous les données à recevoir"
            n226 = case shown="9" w259 {
              tunnel: w258 -> [_ w270 w277 _ _ w285 w296 w304 w312 _ _ _ w320 w328 w336 w344 _ _ _ _ _ _ w353 w362 w371 w379 w389 w396 w407 w416 w424 w434 w441 w451 w459 w468 w477 _ _ _ _ _ _ _ _ _ _ _ _ _ w487 w495 w504 w516 w526]
              tunnel: w260 -> [_ _ _ _ _ w284 _ w303 w311 _ _ _ w319 w327 w335 w343 _ _ _ _ _ _ _ _ _ _ _ _ _ _ _ _ _ _ _ _ _ _ _ _ _ _ _ _ _ _ _ _ _ _ w486 w494 _ _ _]
              frame 0, Default {
              }
              frame 1 {
                n227 = local read "Reception"() -> (w264:string)
                n228 = Type Cast(type=0, x=w270) -> (*(type *) &x=w262:i32)
                n229 = case shown="5, Par défaut" w262 {
                  tunnel: ["OFF" "On_normal" "On_forcé" "On_test" "Etat non défini"] -> w261
                  frame 0 {
                  }
                  frame 1 {
                  }
                  frame 2 {
                  }
                  frame 4 {
                  }
                  frame 5, Default {
                  }
                }
                n230 = call "Date.vi"() -> ("chaîne de date/heure"=w265:string)
                n231 = Concatenate Strings(w264, w265, "  ; " ("chaîne"), "ETAT :" ("chaîne"), w261, "\r") -> (w267:string)
                n232 = local write "Reception"(w267) -> ()
              }
              frame 129 {
                n233 = local read "Reception"() -> (w278:string)
                n234 = Number To Exponential String(number=w277) -> (E-format string=w276:string)  [unwired: 3 in]
                n235 = call "Date.vi"() -> ("chaîne de date/heure"=w279:string)
                n236 = Concatenate Strings(w278, w279, "  ; " ("chaîne"), "Test COM :" ("chaîne"), w276, "\r") -> (w281:string)
                n237 = local write "Reception"(w281) -> ()
              }
              frame 2 {
              }
              frame 3 {
              }
              frame 4 {
                n238 = Number To Decimal String(number=w284) -> (decimal integer string=w288:string)  [unwired: 1 in]
                n239 = Number To Exponential String(number=w285, precision (6)=i16 3 ("précision (6)")) -> (E-format string=w287:string)  [unwired: 2 in]
                n240 = local read "Ana_Battery"() -> (w286:string[][])
                n241 = Build Array(w287, w288) -> (w289:string[])
                n242 = Build Array (concatenate)(w286, w289) -> (w290:string[][])
                n243 = local write "Ana_Battery"(w290) -> ()
              }
              frame 5 {
                n244 = To Byte Integer(number=w296) -> (8bit integer=w293:i8)
                n245 = local read "Reception"() -> (w294:string)
                n246 = case shown="1, Par défaut" w293 {
                  tunnel: ["OK" "Hors intervalle"] -> w292
                  frame 0 {
                  }
                  frame 1, Default {
                  }
                }
                n247 = call "Date.vi"() -> ("chaîne de date/heure"=w295:string)
                n248 = Concatenate Strings(w294, w295, "   ; " ("chaîne"), "ANGLE HORS INTERVALLE :" ("chaîne"), w292, "\r") -> (w298:string)
                n249 = local write "Reception"(w298) -> ()
              }
              frame 6 {
                n250 = Number To Decimal String(number=w303) -> (decimal integer string=w307:string)  [unwired: 1 in]
                n251 = Number To Exponential String(number=w304, precision (6)=i16 3 ("précision (6)")) -> (E-format string=w306:string)  [unwired: 2 in]
                n252 = local read "Other_Angle"() -> (w305:string[][])
                n253 = Build Array(w306, w307) -> (w308:string[])
                n254 = Build Array (concatenate)(w305, w308) -> (w309:string[][])
                n255 = local write "Other_Angle"(w309) -> ()
              }
              frame 7 {
                n256 = Number To Decimal String(number=w311) -> (decimal integer string=w315:string)  [unwired: 1 in]
                n257 = Number To Exponential String(number=w312, precision (6)=i16 3 ("précision (6)")) -> (E-format string=w314:string)  [unwired: 2 in]
                n258 = Build Array(w314, w315) -> (w316:string[])
                n259 = local read "Other_AngularVelocity"() -> (w313:string[][])
                n260 = Build Array (concatenate)(w313, w316) -> (w317:string[][])
                n261 = local write "Other_AngularVelocity"(w317) -> ()
              }
              frame 9 {
              }
              frame 10 {
              }
              frame 11 {
              }
              frame 12 {
                n262 = Number To Decimal String(number=w319) -> (decimal integer string=w323:string)  [unwired: 1 in]
                n263 = Number To Exponential String(number=w320, precision (6)=i16 3 ("précision (6)")) -> (E-format string=w322:string)  [unwired: 2 in]
                n264 = Build Array(w322, w323) -> (w324:string[])
                n265 = local read "Inc_VelocityRightMotor"() -> (w321:string[][])
                n266 = Build Array (concatenate)(w321, w324) -> (w325:string[][])
                n267 = local write "Inc_VelocityRightMotor"(w325) -> ()
              }
              frame 13 {
                n268 = Number To Decimal String(number=w327) -> (decimal integer string=w331:string)  [unwired: 1 in]
                n269 = Number To Exponential String(number=w328, precision (6)=i16 3 ("précision (6)")) -> (E-format string=w330:string)  [unwired: 2 in]
                n270 = Build Array(w330, w331) -> (w332:string[])
                n271 = local read "Inc_VelocityLeftMotor"() -> (w329:string[][])
                n272 = Build Array (concatenate)(w329, w332) -> (w333:string[][])
                n273 = local write "Inc_VelocityLeftMotor"(w333) -> ()
              }
              frame 14 {
                n274 = Number To Decimal String(number=w335) -> (decimal integer string=w339:string)  [unwired: 1 in]
                n275 = Number To Exponential String(number=w336, precision (6)=i16 3 ("précision (6)")) -> (E-format string=w338:string)  [unwired: 2 in]
                n276 = Build Array(w338, w339) -> (w340:string[])
                n277 = local read "Other_Distance"() -> (w337:string[][])
                n278 = Build Array (concatenate)(w337, w340) -> (w341:string[][])
                n279 = local write "Other_Distance"(w341) -> ()
              }
              frame 15 {
                n280 = Number To Decimal String(number=w343) -> (decimal integer string=w347:string)  [unwired: 1 in]
                n281 = Number To Exponential String(number=w344, precision (6)=i16 3 ("précision (6)")) -> (E-format string=w346:string)  [unwired: 2 in]
                n282 = Build Array(w346, w347) -> (w348:string[])
                n283 = local read "Inc_Acceleration"() -> (w345:string[][])
                n284 = Build Array (concatenate)(w345, w348) -> (w349:string[][])
                n285 = local write "Inc_Acceleration"(w349) -> ()
              }
              frame 16 {
              }
              frame 17 {
              }
              frame 18 {
              }
              frame 19 {
              }
              frame 20 {
              }
              frame 21 {
              }
              frame 22 {
                n286 = local read "Reception"() -> (w351:string)
                n287 = Number To Exponential String(number=w353, precision (6)=i16 3 ("précision (6)")) -> (E-format string=w359:string)  [unwired: 2 in]
                n288 = call "Date.vi"() -> ("chaîne de date/heure"=w354:string)
                n289 = Concatenate Strings(w351, w354, "   ; " ("chaîne"), "PRINC_PID_K :" ("chaîne"), w359, "\r") -> (w356:string)
                n290 = local write "Reception"(w356) -> ()
              }
              frame 23 {
                n291 = local read "Reception"() -> (w360:string)
                n292 = Number To Exponential String(number=w362, precision (6)=i16 3 ("précision (6)")) -> (E-format string=w363:string)  [unwired: 2 in]
                n293 = call "Date.vi"() -> ("chaîne de date/heure"=w364:string)
                n294 = Concatenate Strings(w360, w364, "   ; " ("chaîne"), "PRINC_PID_D :" ("chaîne"), w363, "\r") -> (w366:string)
                n295 = local write "Reception"(w366) -> ()
              }
              frame 24 {
                n296 = local read "Reception"() -> (w369:string)
                n297 = Number To Exponential String(number=w371, precision (6)=i16 3 ("précision (6)")) -> (E-format string=w377:string)  [unwired: 2 in]
                n298 = call "Date.vi"() -> ("chaîne de date/heure"=w372:string)
                n299 = Concatenate Strings(w369, w372, "   ; " ("chaîne"), "PRINC_DIR :" ("chaîne"), w377, "\r") -> (w374:string)
                n300 = local write "Reception"(w374) -> ()
              }
              frame 25 {
                n301 = local read "Reception"() -> (w380:string)
                n302 = Number To Exponential String(number=w379, precision (6)=i16 3 ("précision (6)")) -> (E-format string=w386:string)  [unwired: 2 in]
                n303 = call "Date.vi"() -> ("chaîne de date/heure"=w381:string)
                n304 = Concatenate Strings(w380, w381, "   ; " ("chaîne"), "COEF KALMAN :" ("chaîne"), w386, "\r") -> (w383:string)
                n305 = local write "Reception"(w383) -> ()
              }
              frame 26 {
                n306 = local read "Reception"() -> (w387:string)
                n307 = Number To Exponential String(number=w389, precision (6)=i16 3 ("précision (6)")) -> (E-format string=w395:string)  [unwired: 2 in]
                n308 = call "Date.vi"() -> ("chaîne de date/heure"=w390:string)
                n309 = Concatenate Strings(w387, w390, "   ; " ("chaîne"), "ACCELERATION_COEF_FILTRE :" ("chaîne"), w395, "\r") -> (w392:string)
                n310 = local write "Reception"(w392) -> ()
              }
              frame 27 {
                n311 = local read "Reception"() -> (w397:string)
                n312 = Number To Exponential String(number=w396, precision (6)=i16 3 ("précision (6)")) -> (E-format string=w404:string)  [unwired: 2 in]
                n313 = call "Date.vi"() -> ("chaîne de date/heure"=w399:string)
                n314 = Concatenate Strings(w397, w399, "   ; " ("chaîne"), "GUIDON_MAX :" ("chaîne"), w404, "\r") -> (w401:string)
                n315 = local write "Reception"(w401) -> ()
              }
              frame 28 {
                n316 = Number To Exponential String(number=w407, precision (6)=i16 3 ("précision (6)")) -> (E-format string=w408:string)  [unwired: 2 in]
                n317 = local read "Reception"() -> (w405:string)
                n318 = call "Date.vi"() -> ("chaîne de date/heure"=w409:string)
                n319 = Concatenate Strings(w405, w409, "   ; " ("chaîne"), "LIMITE_DISTANCE_UTILISATEUR :" ("chaîne"), w408, "\r") -> (w411:string)
                n320 = local write "Reception"(w411) -> ()
              }
              frame 29 {
                n321 = Number To Exponential String(number=w416, precision (6)=i16 3 ("précision (6)")) -> (E-format string=w422:string)  [unwired: 2 in]
                n322 = local read "Reception"() -> (w414:string)
                n323 = call "Date.vi"() -> ("chaîne de date/heure"=w417:string)
                n324 = Concatenate Strings(w414, w417, "   ; " ("chaîne"), "DEMARRAGE_TOL_ANGLE :" ("chaîne"), w422, "\r") -> (w419:string)
                n325 = local write "Reception"(w419) -> ()
              }
              frame 30 {
                n326 = Number To Exponential String(number=w424, precision (6)=i16 3 ("précision (6)")) -> (E-format string=w431:string)  [unwired: 2 in]
                n327 = local read "Reception"() -> (w423:string)
                n328 = call "Date.vi"() -> ("chaîne de date/heure"=w426:string)
                n329 = Concatenate Strings(w423, w426, "   ; " ("chaîne"), "DEMARRAGE_TOL_GUIDON :" ("chaîne"), w431, "\r") -> (w428:string)
                n330 = local write "Reception"(w428) -> ()
              }
              frame 31 {
                n331 = Number To Exponential String(number=w434, precision (6)=i16 3 ("précision (6)")) -> (E-format string=w440:string)  [unwired: 2 in]
                n332 = local read "Reception"() -> (w432:string)
                n333 = call "Date.vi"() -> ("chaîne de date/heure"=w435:string)
                n334 = Concatenate Strings(w432, w435, "   ; " ("chaîne"), "DEMARRAGE_DELAI_EQUILIBRE :" ("chaîne"), w440, "\r") -> (w437:string)
                n335 = local write "Reception"(w437) -> ()
              }
              frame 32 {
                n336 = Number To Exponential String(number=w441) -> (E-format string=w442:string)  [unwired: 3 in]
                n337 = local read "Reception"() -> (w443:string)
                n338 = call "Date.vi"() -> ("chaîne de date/heure"=w444:string)
                n339 = Concatenate Strings(w443, w444, "   ; " ("chaîne"), "VITESSE_TROTTOIR_MAX :" ("chaîne"), w442, "\r") -> (w446:string)
                n340 = local write "Reception"(w446) -> ()
              }
              frame 33 {
                n341 = Number To Exponential String(number=w451, precision (6)=i16 3 ("précision (6)")) -> (E-format string=w457:string)  [unwired: 2 in]
                n342 = local read "Reception"() -> (w449:string)
                n343 = call "Date.vi"() -> ("chaîne de date/heure"=w452:string)
                n344 = Concatenate Strings(w449, w452, "   ; " ("chaîne"), "POURCENT_SECURITE_MOTEUR :" ("chaîne"), w457, "\r") -> (w454:string)
                n345 = local write "Reception"(w454) -> ()
              }
              frame 34 {
                n346 = Number To Exponential String(number=w459, precision (6)=i16 3 ("précision (6)")) -> (E-format string=w466:string)  [unwired: 2 in]
                n347 = local read "Reception"() -> (w460:string)
                n348 = call "Date.vi"() -> ("chaîne de date/heure"=w461:string)
                n349 = Concatenate Strings(w460, w461, "   ; " ("chaîne"), "COEF_HYSTERISIS :" ("chaîne"), w466, "\r") -> (w463:string)
                n350 = local write "Reception"(w463) -> ()
              }
              frame 35 {
                n351 = Number To Exponential String(number=w468, precision (6)=i16 3 ("précision (6)")) -> (E-format string=w475:string)  [unwired: 2 in]
                n352 = local read "Reception"() -> (w469:string)
                n353 = call "Date.vi"() -> ("chaîne de date/heure"=w470:string)
                n354 = Concatenate Strings(w469, w470, "   ; " ("chaîne"), "COEF_COURANT_1 :" ("chaîne"), w475, "\r") -> (w472:string)
                n355 = local write "Reception"(w472) -> ()
              }
              frame 36 {
                n356 = Number To Exponential String(number=w477, precision (6)=i16 3 ("précision (6)")) -> (E-format string=w484:string)  [unwired: 2 in]
                n357 = local read "Reception"() -> (w478:string)
                n358 = call "Date.vi"() -> ("chaîne de date/heure"=w479:string)
                n359 = Concatenate Strings(w478, w479, "   ; " ("chaîne"), "COEF_COURANT_2 :" ("chaîne"), w484, "\r") -> (w481:string)
                n360 = local write "Reception"(w481) -> ()
              }
              frame 37 {
              }
              frame 38 {
              }
              frame 39 {
              }
              frame 40 {
              }
              frame 41 {
              }
              frame 42 {
              }
              frame 43 {
              }
              frame 44 {
              }
              frame 45 {
              }
              frame 46 {
              }
              frame 47 {
              }
              frame 48 {
              }
              frame 49 {
              }
              frame 50 {
                n361 = Number To Decimal String(number=w486) -> (decimal integer string=w490:string)  [unwired: 1 in]
                n362 = Number To Exponential String(number=w487, precision (6)=i16 3 ("précision (6)")) -> (E-format string=w489:string)  [unwired: 2 in]
                n363 = Build Array(w489, w490) -> (w491:string[])
                n364 = local read "Con_MotorRightTorque"() -> (w488:string[][])
                n365 = Build Array (concatenate)(w488, w491) -> (w492:string[][])
                n366 = local write "Con_MotorRightTorque"(w492) -> ()
              }
              frame 51 {
                n367 = Number To Decimal String(number=w494) -> (decimal integer string=w498:string)  [unwired: 1 in]
                n368 = Number To Exponential String(number=w495, precision (6)=i16 3 ("précision (6)")) -> (E-format string=w497:string)  [unwired: 2 in]
                n369 = Build Array(w497, w498) -> (w499:string[])
                n370 = local read "Con_MotorLeftTorque"() -> (w496:string[][])
                n371 = Build Array (concatenate)(w496, w499) -> (w500:string[][])
                n372 = local write "Con_MotorLeftTorque"(w500) -> ()
              }
              frame 52 {
                n373 = local read "Reception"() -> (w501:string)
                n374 = Type Cast(type=0, x=w504) -> (*(type *) &x=w510:i32)
                n375 = Number To Decimal String(number=w510) -> (decimal integer string=w509:string)  [unwired: 1 in]
                n376 = call "Date.vi"() -> ("chaîne de date/heure"=w503:string)
                n377 = Concatenate Strings(w501, w503, "   ; " ("chaîne"), "ERREUR CARTE COURANT :" ("chaîne"), w509, "\r") -> (w506:string)
                n378 = local write "Reception"(w506) -> ()
              }
              frame 53 {
                n379 = local read "Reception"() -> (w514:string)
                n380 = Type Cast(type=0, x=w516) -> (*(type *) &x=w512:i32)
                n381 = case shown="0, Par défaut" w512 {
                  tunnel: ["Etat à définir" "OK"] -> _
                  frame 0, Default {
                  }
                  frame 1 {
                  }
                }
                n382 = call "Date.vi"() -> ("chaîne de date/heure"=w515:string)
                n383 = Concatenate Strings(w514, w515, "   ; " ("chaîne"), "PRET" ("chaîne"), "" ("chaîne"), "\r") -> (w518:string)
                n384 = local write "Reception"(w518) -> ()
              }
              frame 8 {
                n385 = local read "Reception"() -> (w523:string)
                n386 = Type Cast(type=0, x=w526) -> (*(type *) &x=w532:i32)
                n387 = Number To Decimal String(number=w532) -> (decimal integer string=w531:string)  [unwired: 1 in]
                n388 = call "Date.vi"() -> ("chaîne de date/heure"=w525:string)
                n389 = Concatenate Strings(w523, w525, "   ; " ("chaîne"), "VERBOSE :" ("chaîne"), w531, "\r") -> (w528:string)
                n390 = local write "Reception"(w528) -> ()
              }
            }
          }
        }
      }
    }
  }
  n391 = stacked-sequence {
    tunnel: w9 -> [_ _ _ _ _]
    tunnel: w8 -> [w533 _ _ _ _]
    frame #0 {
      # "Finalisation"
      "Stop main loop" <- w533
    }
    frame #1 {
      n392 = local read "Comm_PortComm"() -> (w536:refnum<visa-resource-name>)
      n393 = local read "error Connexion"() -> (w535:errorcluster)
      n394 = VISA Close(VISA resource name=w536, error in (no error)=w535) -> (error out=w534:errorcluster)
      n395 = local write "error Connexion"(w534) -> ()
    }
    frame #2 {
      n396 = local read "error Connexion"() -> (w539:errorcluster)
      n397 = local read "error"() -> (w538:errorcluster)
      n398 = Merge Errors(w538, w539) -> (w537:errorcluster)
      n399 = call <vilib>:"Simple Error Handler.vi"("error in (no error)"=w537) -> ()  [unwired: 4 in, 5 out]
    }
    frame #3 {
      n400 = Two Button Dialog(message="Save data from reception ?", 1:"Cancel" ("Nom du bouton F (\"Annuler\")")) -> (T button?=w541:bool)  [unwired: 1 in]
      n401 = case shown="Vrai" w541 {
        frame False {
        }
        frame True {
          n402 = local read "Reception"() -> (w544:string)
          n403 = Write to Text File(text=w544) -> (error out=→"sortie d'erreur 3":errorcluster)  [unwired: 3 in, 2 out]
        }
      }
    }
    frame #4 {
      n404 = Two Button Dialog(message="Save physical values ?", 1:"Cancel" ("Nom du bouton F (\"Annuler\")")) -> (T button?=w546:bool)  [unwired: 1 in]
      n405 = case shown="Vrai" w546 {
        frame False {
        }
        frame True {
          n406 = call "Boîte de dialogue utilisateur"() -> ("Angular Velocity"=w548:bool, "Distance"=w549:bool, "Pitch angle"=w550:bool, "Acceleration"=w551:bool, "Left / Right Motor Velocity"=w552:bool, "Battery"=w553:bool, "HandleBar"=w554:bool, "Intensity"=w555:bool, "Left / Right Motor Torque"=w556:bool, "OK"=w557:bool)  [unwired: 9 in, 1 out]
          n407 = case shown="Vrai" w557 {
            tunnel: w556 -> [_ w569]
            tunnel: w555 -> [_ w568]
            tunnel: w554 -> [_ w567]
            tunnel: w553 -> [_ w566]
            tunnel: w552 -> [_ w565]
            tunnel: w551 -> [_ w564]
            tunnel: w550 -> [_ w563]
            tunnel: w549 -> [_ w562]
            tunnel: w548 -> [_ w561]
            frame False {
            }
            frame True {
              n408 = case shown="Vrai" w569 {
                tunnel: w568 -> [_ w591]
                tunnel: w567 -> [_ w590]
                tunnel: w566 -> [_ w589]
                tunnel: w565 -> [_ w588]
                tunnel: w564 -> [_ w587]
                tunnel: w563 -> [_ w586]
                tunnel: w562 -> [_ w585]
                tunnel: w561 -> [_ w584]
                tunnel: [string[][] [] ("Con_MotorLeftTorque") w571] -> w559
                frame False {
                }
                frame True {
                  n409 = local read "Index Tableau"() -> (w580:i32)
                  n410 = local read "Con_MotorRightTorque"() -> (w575:string[][])
                  n411 = local read "Con_MotorLeftTorque"() -> (w583:string[][])
                  n412 = Add(x=w580, y=2) -> (x+y=w577:i32)
                  n413 = local write "Index Tableau"(w577) -> ()
                  n414 = Insert Into Array(array=w583, index (row)=0 ("indice (ligne)"), new element=string[] ["Left Motor Torque", "Time"] ("nouvel élément/sous-tableau")) -> (w576:string[][])  [unwired: 1 in]
                  n415 = Insert Into Array(array=w575, index (row)=0 ("indice (ligne)"), new element=string[] ["Left Motor Torque", "Time"] ("nouvel élément/sous-tableau")) -> (w574:string[][])  [unwired: 1 in]
                  n416 = Insert Into Array(array=w576, index (col)=w577, new element=w574) -> (w578:string[][])  [unwired: 1 in]
                  n417 = case shown="Vrai" w591 {
                    tunnel: w590 -> [_ w609]
                    tunnel: w589 -> [_ w608]
                    tunnel: w588 -> [_ w607]
                    tunnel: w587 -> [_ w606]
                    tunnel: w586 -> [_ w605]
                    tunnel: w585 -> [_ w604]
                    tunnel: w584 -> [_ w603]
                    tunnel: w578 -> [w592 w595]
                    tunnel: [w592 w593] -> w571
                    frame False {
                    }
                    frame True {
                      n418 = local read "Index Tableau"() -> (w598:i32)
                      n419 = local read "Con_Intensity"() -> (w602:string[][])
                      n420 = Add(x=w598, y=2) -> (x+y=w596:i32)
                      n421 = local write "Index Tableau"(w596) -> ()
                      n422 = Insert Into Array(array=w602, index (row)=0 ("indice (ligne)"), new element=string[] ["Intensity", "Time"] ("nouvel élément/sous-tableau")) -> (w594:string[][])  [unwired: 1 in]
                      n423 = Insert Into Array(array=w595, index (col)=w596, new element=w594) -> (w597:string[][])  [unwired: 1 in]
                      n424 = case shown="Vrai" w609 {
                        tunnel: w608 -> [_ w626]
                        tunnel: w607 -> [_ w625]
                        tunnel: w606 -> [_ w624]
                        tunnel: w605 -> [_ w623]
                        tunnel: w604 -> [_ w622]
                        tunnel: w603 -> [_ w621]
                        tunnel: w597 -> [w610 w613]
                        tunnel: [w610 w611] -> w593
                        frame False {
                        }
                        frame True {
                          n425 = local read "Ana_Handlebar"() -> (w616:string[][])
                          n426 = local read "Index Tableau"() -> (w620:i32)
                          n427 = Add(x=w620, y=2) -> (x+y=w615:i32)
                          n428 = local write "Index Tableau"(w615) -> ()
                          n429 = Insert Into Array(array=w616, index (row)=0 ("indice (ligne)"), new element=string[] ["HandleBar", "Time"] ("nouvel élément/sous-tableau")) -> (w612:string[][])  [unwired: 1 in]
                          n430 = Insert Into Array(array=w613, index (col)=w615, new element=w612) -> (w614:string[][])  [unwired: 1 in]
                          n431 = case shown="Vrai" w626 {
                            tunnel: w625 -> [_ w642]
                            tunnel: w624 -> [_ w641]
                            tunnel: w623 -> [_ w640]
                            tunnel: w622 -> [_ w639]
                            tunnel: w621 -> [_ w638]
                            tunnel: w614 -> [w627 w629]
                            tunnel: [w627 w628] -> w611
                            frame False {
                            }
                            frame True {
                              n432 = local read "Ana_Battery"() -> (w636:string[][])
                              n433 = local read "Index Tableau"() -> (w632:i32)
                              n434 = Add(x=w632, y=2) -> (x+y=w637:i32)
                              n435 = local write "Index Tableau"(w637) -> ()
                              n436 = Insert Into Array(array=w636, index (row)=0 ("indice (ligne)"), new element=string[] ["Battery", "Time"] ("nouvel élément/sous-tableau")) -> (w630:string[][])  [unwired: 1 in]
                              n437 = Insert Into Array(array=w629, index (col)=w637, new element=w630) -> (w631:string[][])  [unwired: 1 in]
                              n438 = case shown="Vrai" w642 {
                                tunnel: w641 -> [_ w664]
                                tunnel: w640 -> [_ w663]
                                tunnel: w639 -> [_ w662]
                                tunnel: w638 -> [_ w661]
                                tunnel: w631 -> [w643 w647]
                                tunnel: [w643 w644] -> w628
                                frame False {
                                }
                                frame True {
                                n439 = local read "Index Tableau"() -> (w656:i32)
                                n440 = local read "Inc_VelocityLeftMotor"() -> (w660:string[][])
                                n441 = local read "Inc_VelocityLeftMotor"() -> (w652:string[][])
                                n442 = Add(x=w656, y=2) -> (x+y=w650:i32)
                                n443 = Add(x=w650, y=2) -> (x+y=w651:i32)
                                n444 = Insert Into Array(array=w660, index (row)=0 ("indice (ligne)"), new element=string[] ["Left Motor  Velocity", "Time"] ("nouvel élément/sous-tableau")) -> (w646:string[][])  [unwired: 1 in]
                                n445 = local write "Index Tableau"(w651) -> ()
                                n446 = Insert Into Array(array=w647, index (col)=w650, new element=w646) -> (w648:string[][])  [unwired: 1 in]
                                n447 = Insert Into Array(array=w652, index (row)=0 ("indice (ligne)"), new element=string[] ["Right Motor Velocity", "Time"] ("nouvel élément/sous-tableau")) -> (w649:string[][])  [unwired: 1 in]
                                n448 = Insert Into Array(array=w648, index (col)=w651, new element=w649) -> (w645:string[][])  [unwired: 1 in]
                                n449 = case shown="Vrai" w664 {
                                tunnel: w663 -> [_ w678]
                                tunnel: w662 -> [_ w677]
                                tunnel: w661 -> [_ w676]
                                tunnel: w645 -> [w665 w669]
                                tunnel: [w665 w666] -> w644
                                frame False {
                                }
                                frame True {
                                n450 = local read "Inc_Acceleration"() -> (w675:string[][])
                                n451 = local read "Index Tableau"() -> (w671:i32)
                                n452 = Add(x=w671, y=2) -> (x+y=w667:i32)
                                n453 = Insert Into Array(array=w675, index (row)=0 ("indice (ligne)"), new element=string[] ["Acceleration", "Time"] ("nouvel élément/sous-tableau")) -> (w670:string[][])  [unwired: 1 in]
                                n454 = local write "Index Tableau"(w667) -> ()
                                n455 = Insert Into Array(array=w669, index (col)=w667, new element=w670) -> (w668:string[][])  [unwired: 1 in]
                                n456 = case shown="Vrai" w678 {
                                tunnel: w677 -> [_ w691]
                                tunnel: w676 -> [_ w690]
                                tunnel: w668 -> [w679 w683]
                                tunnel: [w679 w680] -> w666
                                frame False {
                                }
                                frame True {
                                n457 = local read "Other_Angle"() -> (w684:string[][])
                                n458 = local read "Index Tableau"() -> (w688:i32)
                                n459 = Add(x=w688, y=2) -> (x+y=w681:i32)
                                n460 = Insert Into Array(array=w684, index (row)=0 ("indice (ligne)"), new element=string[] ["Angle", "Time"] ("nouvel élément/sous-tableau")) -> (w689:string[][])  [unwired: 1 in]
                                n461 = local write "Index Tableau"(w681) -> ()
                                n462 = Insert Into Array(array=w683, index (col)=w681, new element=w689) -> (w682:string[][])  [unwired: 1 in]
                                n463 = case shown="Vrai" w691 {
                                tunnel: w690 -> [_ w703]
                                tunnel: w682 -> [w692 w695]
                                tunnel: [w692 w693] -> w680
                                frame False {
                                }
                                frame True {
                                n464 = local read "Other_Distance"() -> (w702:string[][])
                                n465 = local read "Index Tableau"() -> (w698:i32)
                                n466 = Add(x=w698, y=2) -> (x+y=w696:i32)
                                n467 = Insert Into Array(array=w702, index (row)=0 ("indice (ligne)"), new element=string[] ["Distance", "Time"] ("nouvel élément/sous-tableau")) -> (w697:string[][])  [unwired: 1 in]
                                n468 = local write "Index Tableau"(w696) -> ()
                                n469 = Insert Into Array(array=w695, index (col)=w696, new element=w697) -> (w694:string[][])  [unwired: 1 in]
                                n470 = case shown="Vrai" w703 {
                                tunnel: w694 -> [w704 w706]
                                tunnel: [w704 w705] -> w693
                                frame False {
                                }
                                frame True {
                                n471 = local read "Index Tableau"() -> (w711:i32)
                                n472 = local read "Other_AngularVelocity"() -> (w707:string[][])
                                n473 = Add(x=w711, y=2) -> (x+y=w713:i32)
                                n474 = local write "Index Tableau"(w713) -> ()
                                n475 = Insert Into Array(array=w707, index (row)=0 ("indice (ligne)"), new element=string[] ["AngularVelocity", "Time"] ("nouvel élément/sous-tableau")) -> (w712:string[][])  [unwired: 1 in]
                                n476 = Insert Into Array(array=w706, index (col)=w713, new element=w712) -> (w705:string[][])  [unwired: 1 in]
                                }
                                }
                                }
                                }
                                }
                                }
                                }
                                }
                                }
                              }
                            }
                          }
                        }
                      }
                    }
                  }
                }
              }
              n477 = call-poly <vilib>:"Write To Spreadsheet File.vi"("delimiter (\\t)"=";" ("delimiter (\\t)"), "2D data"=w559) -> ()  [unwired: 6 in, 1 out]
              "Index Tableau" <- 0 ("Index Tableau")
            }
          }
        }
      }
    }
  }
  n478 = flat-sequence {
    tunnel: w6 -> [w716]
    tunnel: w1 -> [w714]
    frame #0 {
      n479 = Tick Count (ms)() -> (millisecond timer value=w718:u32)
      n480 = Subtract(x=w718, y=w714) -> (x-y=w717:u32)
      n481 = Divide(x=w717, y=w716) -> (x/y=→"Frequency":dbl)
    }
  }
